vi "Begin.vi"(8 "error in":errorcluster) -> (0 "error out":errorcluster)   [LabVIEW 2016]
doc: "Called before other user functions, this VI is expected to open initial I/O refnums, load in file data, and do all program initialization. Notice that the <B>error out</B> terminal is simply used for data flow. Wiring it to other structures or subVIs ensures that this VI runs first."
uses:
  <vilib>/Rock Robotics/WPI/DriverStation/WPI_DriverStationRobotMode2.ctl
  <vilib>/Rock Robotics/WPI/Joystick/WPI_JoystickDeviceEnum.ctl
  <vilib>/Rock Robotics/WPI/ThirdParty/CanMotor/TalonSRX/WPI_CANTalonSRX_APIControlMode.ctl
  <vilib>/Rock Robotics/SystemInterfaces/DIO/FPGA_DIOPWMChannel.ctl
  <vilib>/Rock Robotics/WPI/Solenoid/WPI_SolenoidChannel.ctl
  <vilib>/Rock Robotics/WPI/ThirdParty/CanMotor/TalonSRX/WPI_CANTalonSRX_APIFeedbackSelect.ctl
  <vilib>/Rock Robotics/WPI/SafetyOutput/WPI_SafetyOutputConfigMenu.ctl
  <vilib>/Rock Robotics/SystemInterfaces/DIO/FPGA_DIOChannel.ctl
  <vilib>/Rock Robotics/SystemInterfaces/spilib/spi_bus.ctl
  Robot Global Data.vi
  <vilib>/Rock Robotics/Network Tables/NT Write String Array.vi
  <vilib>/Rock Robotics/WPI/MotorControl/WPI_MotorControlOpen VictorSP.vi
  <vilib>/Rock Robotics/WPI/Solenoid/WPI_SolenoidOpenDouble.vi
  <vilib>/Rock Robotics/WPI/Switch/WPI_SwitchOpenLimit.vi
  <vilib>/Rock Robotics/Network Tables/NT Write Boolean.vi
  <vilib>/Rock Robotics/WPI/Gyro/WPI_GyroXRS450_SPI_Open.vi
  <vilib>/Rock Robotics/WPI/Counter/WPI_CounterDigitalInputToDigitalSource.vi
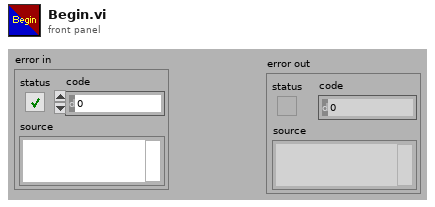
[diagram p1: front panel]
types:
  T1 = typedef "FPGA_DIOChannel.ctl" = enum8{"DIO 0", "DIO 1", "DIO 2", "DIO 3", "DIO 4", "DIO 5", "DIO 6", "DIO 7", "DIO 8", "DIO 9", "DIO MXP 0", "DIO MXP 1", "DIO MXP 2", "DIO MXP 3", "DIO MXP 4", "DIO MXP 5", "DIO MXP 6", "DIO MXP 7", "DIO MXP 8", "DIO MXP 9", "DIO MXP 10", "DIO MXP 11", "DIO MXP 12", "DIO MXP 13", "DIO MXP 14", "DIO MXP 15", "SPI Port CS1", "SPI Port CS2", "SPI Port CS3", "SPI Port MISO", "SPI Port MOSI", "Invalid"}
  T2 = typedef "spi_bus.ctl" = enum16{"SPI On-Board, CS0", "SPI On-Board, CS1", "SPI On-Board, CS2", "SPI On-Board, CS3", "SPI MXP", "Invalid"}
  T3 = typedef "WPI_CANTalonSRX_APIControlMode.ctl" = enum8{"Percent VBus", "Speed", "Position", "Slave", "Unchanged / Invalid", "Voltage Compensation", "Current", "Motion Profile", "Motion Magic"}
  T4 = typedef "WPI_JoystickDeviceEnum.ctl" = enum16{"USB 0", "USB 1", "USB 2", "USB 3", "USB 4", "USB 5"}
  T5 = typedef "WPI_SafetyOutputConfigMenu.ctl" = enum16{"Enable", "Disable"}
  T6 = typedef "WPI_SolenoidChannel.ctl" = enum8{"Solenoid 0", "Solenoid 1", "Solenoid 2", "Solenoid 3", "Solenoid 4", "Solenoid 5", "Solenoid 6", "Solenoid 7", "Invalid"}
  T7 = typedef "WPI_CANTalonSRX_APIFeedbackSelect.ctl" = enum16{"Digital Quadrature Encoder", "Analog Potentiometer", "Analog Encoder", "Count on Quad-A (Rising-Edge)", "Count on Quad-A (Falling-Edge)", "CTR Magnetic Enc (Absolute)", "CTR Magnetic Enc (Relative)", "Pulse Width"}
  T8 = typedef "FPGA_DIOPWMChannel.ctl" = enum8{"PWM 0", "PWM 1", "PWM 2", "PWM 3", "PWM 4", "PWM 5", "PWM 6", "PWM 7", "PWM 8", "PWM 9", "PWM MXP 0", "PWM MXP 1", "PWM MXP 2", "PWM MXP 3", "PWM MXP 4", "PWM MXP 5", "PWM MXP 6", "PWM MXP 7", "PWM MXP 8", "PWM MXP 9", "Invalid"}
  T9 = typedef "WPI_DriverStationRobotMode2.ctl" = enum16{"Autonomous Disabled", "Autonomous Enabled", "Teleop Disabled", "Teleop Enabled", "Disconnected", "Finish", "Test Disabled", "Test Enabled", "Emergency Stopped"}
  T10 = typedef "WPI_JoystickDevRef.ctl" = cluster{"Device":T4}
  T11 = typedef "WPI_DigitalInputDevRef.ctl" = cluster{"DevStatus":errorcluster, "DIO Channel":T1}
  T12 = typedef "FPGA_CounterEncoderSourceConvertionLVSourceType.ctl" = cluster{"DevStatus":errorcluster, "AnalogTriggerMode?":bool, "DigitalMode":cluster{"DIO Channel":T13}, "AnalogTriggerMode":cluster{"AnalogTriggerIndex":T14, "OutputType":T15}}
  T13 = typedef "FPGA_DIODigitalSourceChannel.ctl" = enum8{"DIO 0", "DIO 1", "DIO 2", "DIO 3", "DIO 4", "DIO 5", "DIO 6", "DIO 7", "DIO 8", "DIO 9", "DIO MXP 0", "DIO MXP 1", "DIO MXP 2", "DIO MXP 3", "DIO MXP 4", "DIO MXP 5", "DIO MXP 6", "DIO MXP 7", "DIO MXP 8", "DIO MXP 9", "DIO MXP 10", "DIO MXP 11", "DIO MXP 12", "DIO MXP 13", "DIO MXP 14", "DIO MXP 15", "Disabled"}
  T14 = typedef "FPGA_AnalogTriggerIndex.ctl" = enum8{"Trig 0", "Trig 1", "Trig 2", "Trig 3", "Trig 4", "Trig 5", "Trig 6", "Trig 7", "Invalid"}
  T15 = typedef "FPGA_AnalogTriggerOutType.ctl" = enum16{"InWindow", "TriggerState", "Rising", "Falling"}
  T16 = typedef "WPI_EncoderDevRef.ctl" = cluster{"DevStatus":errorcluster, "EncoderIndex":T17, "CounterIndex":T18, "DistancePerCount":dbl, "Decoding Type":T19}
  T17 = typedef "FPGA_EncoderIdx.ctl" = enum8{"Enc 0", "Enc 1", "Enc 2", "Enc 3", "Enc 4", "Enc 5", "Enc 6", "Enc 7", "Invalid"}
  T18 = typedef "FPGA_CounterCtrSystemIndex.ctl" = enum8{"Ctr 0", "Ctr 1", "Ctr 2", "Ctr 3", "Ctr 4", "Ctr 5", "Ctr 6", "Ctr 7", "Invalid"}
  T19 = typedef "WPI_EncoderType.ctl" = enum16{"1x", "2x", "4x"}
  T20 = typedef "WPI_SolenoidDevRef.ctl" = cluster{"DevStatus":errorcluster, "Pneumatics Control Module":u8, "Forward Solenoid Channel":T6, "Reverse Solenoid Channel":T6}
  T21 = typedef "WPI_MotorControlDeviceRef.ctl" = cluster{"DeviceStatus":errorcluster, "Type":T22, "PWM":cluster{"PWM Channel":T8, "DeadBand":T23}, "CAN":cluster{"Device Number":u8, "SetOutput VI Ref":variant, "GetOutput VI Ref":variant, "Enable VI Ref":variant, "Disable VI Ref":variant, "Data":variant}, "Invert":bool}
  T22 = typedef "WPI_MotorControlType.ctl" = enum16{"PWM", "CAN"}
  T23 = typedef "WPI_PWMDeadband.ctl" = cluster{"Name":string, "maxPositivePwm":i32, "minPositivePwm":i32, "centerPwm":i32, "maxNegativePwm":i32, "minNegativePwm":i32, "angularRange":u16}
  T24 = typedef "WPI_SwitchDevRef.ctl" = cluster{"DevStatus":errorcluster, "DIO Channel":T1, "CntIndex":T18, "Normally Closed":bool}
  T25 = typedef "WPI_GyroDevRef.ctl" = cluster{"DevStatus":errorcluster, "Analog Channel":T26, "Offset":dbl, "Gain (VoltsPerDegree/Second)":dbl, "Gyro Type":enum16{"Analog", "XRS450"}, "Handle":i32, "SPI Bus":T2, "Device Found":bool, "Sample Rate":dbl, "Calibrate On Open":bool}
  T26 = typedef "FPGA_AIChannel.ctl" = enum8{"AI 0", "AI 1", "AI 2", "AI 3", "AI MXP 0", "AI MXP 1", "AI MXP 2", "AI MXP 3", "Invalid"}
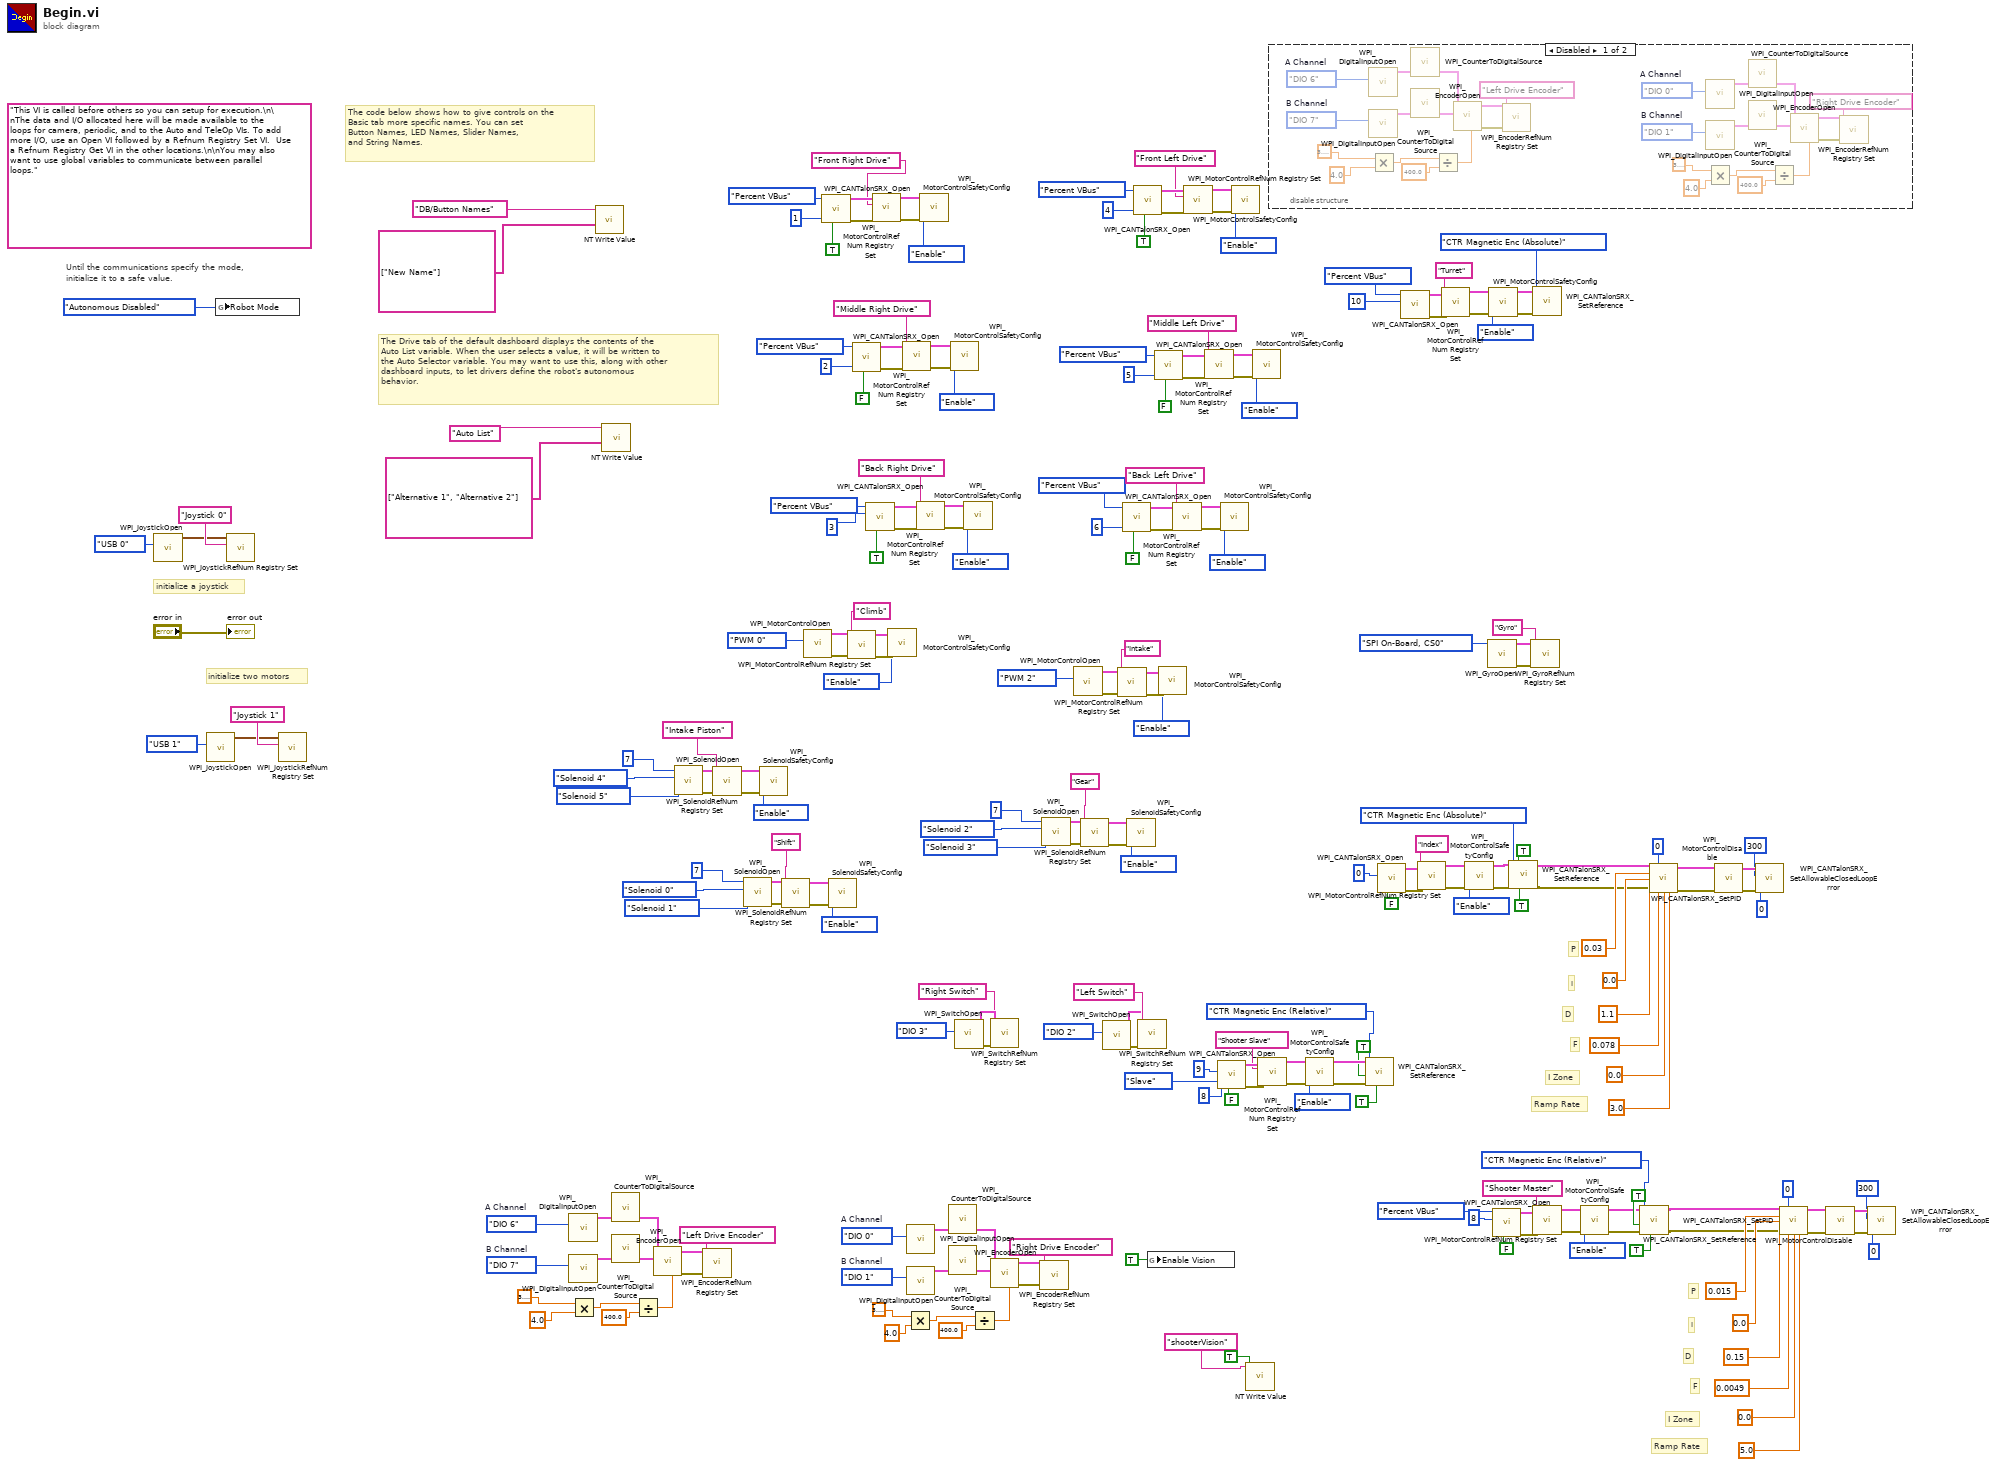
[diagram p0: block diagram]
diagram:
  w19 = FPGA_DIOChannel."DIO 1"  # B Channel
  w18 = FPGA_DIOChannel."DIO 0"  # A Channel
  w28 = FPGA_DIOChannel."DIO 7"  # B Channel
  w27 = FPGA_DIOChannel."DIO 6"  # A Channel
  (unwired) "This VI is called before others so you can setup for execution.\n\nThe data and I/O allocated here will be made available to the loops for camera, periodic, and to the Auto and TeleOp VIs. To add more I/O, use an Open VI followed by a Refnum Registry Set VI.  Use a Refnum Registry Get VI in the other locations.\n\nYou may also want to use global variables to communicate between parallel loops."
  # "Ramp Rate"
  # "I Zone"
  # "F"
  # "D"
  # "I"
  # "P"
  # "Ramp Rate"
  # "I Zone"
  # "F"
  # "D"
  # "I"
  # "P"
  # "initialize two motors"
  # "The Drive tab of the default dashboard displays the contents of the\nAuto List variable. When the user selects a value, it will be written to\nthe Auto Selector variable. You may want to use this, along with other\ndashboard inputs, to let drivers define the robot's autonomous\nbehavior."
  # "The code below shows how to give controls on the\nBasic tab more specific names. You can set\nButton Names, LED Names, Slider Names,\nand String Names."
  # "initialize a joystick"
  # "Until the communications specify the mode,\ninitialize it to a safe value."
  n1 = call <vilib>:"WPI_JoystickOpen.vi"("JoystickDevice"=WPI_JoystickDeviceEnum."USB 0") -> ("JoystickDevRef"=w231:T10)  [unwired: 10 in]
  n2 = call <vilib>:"WPI_JoystickOpen.vi"("JoystickDevice"=WPI_JoystickDeviceEnum."USB 1") -> ("JoystickDevRef"=w78:T10)  [unwired: 10 in]
  n3 = global write "Robot Global Data.vi" "Robot Mode"(WPI_DriverStationRobotMode2."Autonomous Disabled" ("Robot Mode")) -> ()
  n4 = call <vilib>:"WPI_JoystickRefNum Registry Set.vi"("refnum name"="Joystick 0", "JoystickDevRef"=w231) -> ()  [unwired: 8 in, 2 out]
  n5 = call <vilib>:"WPI_JoystickRefNum Registry Set.vi"("refnum name"="Joystick 1", "JoystickDevRef"=w78) -> ()  [unwired: 8 in, 2 out]
  n6 = call <vilib>:"WPI_DigitalInputOpen.vi"("DIO Channel"=w27) -> ("DigitalInputDevRef"=w24:T11)  [unwired: 1 in, 9 out]
  n7 = call <vilib>:"WPI_DigitalInputOpen.vi"("DIO Channel"=w28) -> ("DigitalInputDevRef"=w25:T11)  [unwired: 1 in, 9 out]
  n8 = Multiply(x=3.141592653589793, y=4.0) -> (x*y=w3:dbl)
  n9 = call-poly <vilib>:"NT Write Value.vi"("String Array"=string[] ["New Name"], "Name"="DB/Button Names") -> ()  [unwired: 9 in, 1 out]
  n10 = call-poly <vilib>:"NT Write Value.vi"("String Array"=string[] ["Alternative 1", "Alternative 2"], "Name"="Auto List") -> ()  [unwired: 9 in, 1 out]
  n11 = call-poly <vilib>:"WPI_CounterToDigitalSource.vi"("DigitalInputDevRef"=w24) -> ("Digital Source"=w23:T12)  [unwired: 6 out]
  n12 = call-poly <vilib>:"WPI_CounterToDigitalSource.vi"("DigitalInputDevRef"=w25) -> ("Digital Source"=w26:T12)  [unwired: 6 out]
  n13 = Divide(x=w3, y=400.0) -> (x/y=w1:dbl)
  n14 = call <vilib>:"WPI_EncoderOpen.vi"("DistancePerCount"=w1, "BSource"=w26, "ASource"=w23) -> ("error out"=w22:errorcluster, "EncoderDevRef"=w21:T16)  [unwired: 5 in, 2 out]
  n15 = call-poly <vilib>:"WPI_SolenoidOpen.vi"("Reverse Solenoid Channel"=WPI_SolenoidChannel."Solenoid 5", "Forward Solenoid Channel"=WPI_SolenoidChannel."Solenoid 4", "Pneumatics Control Module (0)"=u8 7) -> ("error out"=w155:errorcluster, "SolenoidDevRef"=w154:T20)  [unwired: 7 in]
  n16 = call <vilib>:"WPI_EncoderRefNum Registry Set.vi"("error in (no error)"=w22, "refnum name"="Left Drive Encoder", "EncoderDevRef"=w21) -> ()  [unwired: 7 in, 2 out]
  n17 = call <vilib>:"WPI_SolenoidRefNum Registry Set.vi"("error in (no error)"=w155, "refnum name"="Intake Piston", "SolenoidDevRef"=w154) -> ("error out"=w152:errorcluster, "SolenoidDevRef"=w151:T20)  [unwired: 7 in]
  n18 = call-poly <vilib>:"WPI_SolenoidOpen.vi"("Reverse Solenoid Channel"=WPI_SolenoidChannel."Solenoid 1", "Forward Solenoid Channel"=WPI_SolenoidChannel."Solenoid 0", "Pneumatics Control Module (0)"=u8 7) -> ("error out"=w85:errorcluster, "SolenoidDevRef"=w84:T20)  [unwired: 7 in]
  n19 = call <vilib>:"WPI_SolenoidSafetyConfig.vi"("error in (no error)"=w152, "mode"=WPI_SafetyOutputConfigMenu."Enable", "SolenoidDevRef"=w151) -> ()  [unwired: 7 in, 2 out]
  n20 = call <vilib>:"WPI_SolenoidRefNum Registry Set.vi"("error in (no error)"=w85, "refnum name"="Shift", "SolenoidDevRef"=w84) -> ("error out"=w82:errorcluster, "SolenoidDevRef"=w81:T20)  [unwired: 7 in]
  n21 = call-poly <vilib>:"WPI_MotorControlOpen.vi"("PWM Channel"=FPGA_DIOPWMChannel."PWM 0") -> ("error out"=w170:errorcluster, "MotorControlDeviceRef"=w169:T21)  [unwired: 9 in]
  n22 = call <vilib>:"WPI_CANTalonSRX_Open.vi"("Invert"=TRUE, "Device Number"=u8 1, "Control Mode"=WPI_CANTalonSRX_APIControlMode."Percent VBus") -> ("error out"=w186:errorcluster, "CAN Talon SRX Ref"=w185:T21)  [unwired: 7 in]
  n23 = call <vilib>:"WPI_SolenoidSafetyConfig.vi"("error in (no error)"=w82, "mode"=WPI_SafetyOutputConfigMenu."Enable", "SolenoidDevRef"=w81) -> ()  [unwired: 7 in, 2 out]
  n24 = call <vilib>:"WPI_MotorControlRefNum Registry Set.vi"("error in (no error)"=w170, "refnum name"="Climb", "MotorControlDevRef"=w169) -> ("error out"=w166:errorcluster, "MotorControlDevRef"=w165:T21)  [unwired: 7 in]
  n25 = call <vilib>:"WPI_CANTalonSRX_Open.vi"("Invert"=FALSE, "Device Number"=u8 2, "Control Mode"=WPI_CANTalonSRX_APIControlMode."Percent VBus") -> ("error out"=w221:errorcluster, "CAN Talon SRX Ref"=w220:T21)  [unwired: 7 in]
  n26 = call <vilib>:"WPI_CANTalonSRX_Open.vi"("Invert"=TRUE, "Device Number"=u8 3, "Control Mode"=WPI_CANTalonSRX_APIControlMode."Percent VBus") -> ("error out"=w204:errorcluster, "CAN Talon SRX Ref"=w203:T21)  [unwired: 7 in]
  n27 = call <vilib>:"WPI_MotorControlRefNum Registry Set.vi"("error in (no error)"=w186, "refnum name"="Front Right Drive", "MotorControlDevRef"=w185) -> ("error out"=w184:errorcluster, "MotorControlDevRef"=w183:T21)  [unwired: 7 in]
  n28 = call <vilib>:"WPI_MotorControlSafetyConfig.vi"("error in (no error)"=w166, "mode"=WPI_SafetyOutputConfigMenu."Enable", "MotorControlDevRef"=w165) -> ()  [unwired: 7 in, 2 out]
  n29 = call <vilib>:"WPI_MotorControlRefNum Registry Set.vi"("error in (no error)"=w221, "refnum name"="Middle Right Drive", "MotorControlDevRef"=w220) -> ("error out"=w219:errorcluster, "MotorControlDevRef"=w218:T21)  [unwired: 7 in]
  n30 = call <vilib>:"WPI_DigitalInputOpen.vi"("DIO Channel"=w18) -> ("DigitalInputDevRef"=w15:T11)  [unwired: 1 in, 9 out]
  n31 = call <vilib>:"WPI_DigitalInputOpen.vi"("DIO Channel"=w19) -> ("DigitalInputDevRef"=w16:T11)  [unwired: 1 in, 9 out]
  n32 = Multiply(x=3.141592653589793, y=4.0) -> (x*y=w8:dbl)
  n33 = call <vilib>:"WPI_MotorControlRefNum Registry Set.vi"("error in (no error)"=w204, "refnum name"="Back Right Drive", "MotorControlDevRef"=w203) -> ("error out"=w202:errorcluster, "MotorControlDevRef"=w201:T21)  [unwired: 7 in]
  n34 = call <vilib>:"WPI_MotorControlSafetyConfig.vi"("error in (no error)"=w184, "mode"=WPI_SafetyOutputConfigMenu."Enable", "MotorControlDevRef"=w183) -> ()  [unwired: 7 in, 2 out]
  n35 = call-poly <vilib>:"WPI_CounterToDigitalSource.vi"("DigitalInputDevRef"=w15) -> ("Digital Source"=w14:T12)  [unwired: 6 out]
  n36 = call-poly <vilib>:"WPI_CounterToDigitalSource.vi"("DigitalInputDevRef"=w16) -> ("Digital Source"=w17:T12)  [unwired: 6 out]
  n37 = call <vilib>:"WPI_MotorControlSafetyConfig.vi"("error in (no error)"=w219, "mode"=WPI_SafetyOutputConfigMenu."Enable", "MotorControlDevRef"=w218) -> ()  [unwired: 7 in, 2 out]
  n38 = call-poly <vilib>:"WPI_SwitchOpen.vi"("DIO Channel"=FPGA_DIOChannel."DIO 3") -> ("error out"=w76:errorcluster, "SwitchDevRef"=w75:T24)  [unwired: 9 in]
  n39 = call <vilib>:"WPI_MotorControlSafetyConfig.vi"("error in (no error)"=w202, "mode"=WPI_SafetyOutputConfigMenu."Enable", "MotorControlDevRef"=w201) -> ()  [unwired: 7 in, 2 out]
  n40 = Divide(x=w8, y=400.0) -> (x/y=w6:dbl)
  n41 = call <vilib>:"WPI_SwitchRefNum Registry Set.vi"("error in (no error)"=w76, "refnum name"="Right Switch", "SwitchDevRef"=w75) -> ()  [unwired: 7 in, 2 out]
  n42 = call <vilib>:"WPI_EncoderOpen.vi"("DistancePerCount"=w6, "BSource"=w17, "ASource"=w14) -> ("error out"=w13:errorcluster, "EncoderDevRef"=w12:T16)  [unwired: 5 in, 2 out]
  n43 = call <vilib>:"WPI_EncoderRefNum Registry Set.vi"("error in (no error)"=w13, "refnum name"="Right Drive Encoder", "EncoderDevRef"=w12) -> ()  [unwired: 7 in, 2 out]
  n44 = call-poly <vilib>:"WPI_SolenoidOpen.vi"("Reverse Solenoid Channel"=WPI_SolenoidChannel."Solenoid 3", "Forward Solenoid Channel"=WPI_SolenoidChannel."Solenoid 2", "Pneumatics Control Module (0)"=u8 7) -> ("error out"=w142:errorcluster, "SolenoidDevRef"=w143:T20)  [unwired: 7 in]
  n45 = call-poly <vilib>:"WPI_MotorControlOpen.vi"("PWM Channel"=FPGA_DIOPWMChannel."PWM 2") -> ("error out"=w164:errorcluster, "MotorControlDeviceRef"=w163:T21)  [unwired: 9 in]
  n46 = call <vilib>:"WPI_SolenoidRefNum Registry Set.vi"("error in (no error)"=w142, "refnum name"="Gear", "SolenoidDevRef"=w143) -> ("error out"=w145:errorcluster, "SolenoidDevRef"=w146:T20)  [unwired: 7 in]
  n47 = call-poly <vilib>:"WPI_SwitchOpen.vi"("DIO Channel"=FPGA_DIOChannel."DIO 2") -> ("error out"=w69:errorcluster, "SwitchDevRef"=w70:T24)  [unwired: 9 in]
  n48 = call <vilib>:"WPI_MotorControlRefNum Registry Set.vi"("error in (no error)"=w164, "refnum name"="Intake", "MotorControlDevRef"=w163) -> ("error out"=w160:errorcluster, "MotorControlDevRef"=w159:T21)  [unwired: 7 in]
  n49 = call <vilib>:"WPI_CANTalonSRX_Open.vi"("Invert"=FALSE, "Device Number"=u8 6, "Control Mode"=WPI_CANTalonSRX_APIControlMode."Percent VBus") -> ("error out"=w196:errorcluster, "CAN Talon SRX Ref"=w195:T21)  [unwired: 7 in]
  n50 = call <vilib>:"WPI_SolenoidSafetyConfig.vi"("error in (no error)"=w145, "mode"=WPI_SafetyOutputConfigMenu."Enable", "SolenoidDevRef"=w146) -> ()  [unwired: 7 in, 2 out]
  n51 = call <vilib>:"WPI_CANTalonSRX_Open.vi"("Invert"=TRUE, "Device Number"=u8 4, "Control Mode"=WPI_CANTalonSRX_APIControlMode."Percent VBus") -> ("error out"=w212:errorcluster, "CAN Talon SRX Ref"=w211:T21)  [unwired: 7 in]
  n52 = call <vilib>:"WPI_SwitchRefNum Registry Set.vi"("error in (no error)"=w69, "refnum name"="Left Switch", "SwitchDevRef"=w70) -> ()  [unwired: 7 in, 2 out]
  n53 = global write "Robot Global Data.vi" "Enable Vision"(TRUE ("Enable Vision")) -> ()
  n54 = call <vilib>:"WPI_CANTalonSRX_Open.vi"("Invert"=FALSE, "Device Number"=u8 5, "Control Mode"=WPI_CANTalonSRX_APIControlMode."Percent VBus") -> ("error out"=w178:errorcluster, "CAN Talon SRX Ref"=w173:T21)  [unwired: 7 in]
  n55 = call <vilib>:"WPI_MotorControlSafetyConfig.vi"("error in (no error)"=w160, "mode"=WPI_SafetyOutputConfigMenu."Enable", "MotorControlDevRef"=w159) -> ()  [unwired: 7 in, 2 out]
  n56 = call <vilib>:"WPI_MotorControlRefNum Registry Set.vi"("error in (no error)"=w196, "refnum name"="Back Left Drive", "MotorControlDevRef"=w195) -> ("error out"=w194:errorcluster, "MotorControlDevRef"=w193:T21)  [unwired: 7 in]
  n57 = call <vilib>:"WPI_MotorControlRefNum Registry Set.vi"("error in (no error)"=w212, "refnum name"="Front Left Drive", "MotorControlDevRef"=w211) -> ("error out"=w210:errorcluster, "MotorControlDevRef"=w209:T21)  [unwired: 7 in]
  n58 = call <vilib>:"WPI_MotorControlRefNum Registry Set.vi"("error in (no error)"=w178, "refnum name"="Middle Left Drive", "MotorControlDevRef"=w173) -> ("error out"=w177:errorcluster, "MotorControlDevRef"=w176:T21)  [unwired: 7 in]
  n59 = call <vilib>:"WPI_CANTalonSRX_Open.vi"("Invert"=FALSE, "Master Device Number"=u8 8, "Device Number"=u8 9, "Control Mode"=WPI_CANTalonSRX_APIControlMode."Slave") -> ("error out"=w117:errorcluster, "CAN Talon SRX Ref"=w118:T21)  [unwired: 6 in]
  n60 = call <vilib>:"WPI_MotorControlSafetyConfig.vi"("error in (no error)"=w194, "mode"=WPI_SafetyOutputConfigMenu."Enable", "MotorControlDevRef"=w193) -> ()  [unwired: 7 in, 2 out]
  n61 = call <vilib>:"WPI_MotorControlSafetyConfig.vi"("error in (no error)"=w210, "mode"=WPI_SafetyOutputConfigMenu."Enable", "MotorControlDevRef"=w209) -> ()  [unwired: 7 in, 2 out]
  n62 = call-poly <vilib>:"NT Write Value.vi"("Boolean"=TRUE, "Name"="shooterVision") -> ()  [unwired: 9 in, 1 out]
  n63 = call <vilib>:"WPI_MotorControlSafetyConfig.vi"("error in (no error)"=w177, "mode"=WPI_SafetyOutputConfigMenu."Enable", "MotorControlDevRef"=w176) -> ()  [unwired: 7 in, 2 out]
  n64 = call <vilib>:"WPI_MotorControlRefNum Registry Set.vi"("error in (no error)"=w117, "refnum name"="Shooter Slave", "MotorControlDevRef"=w118) -> ("error out"=w113:errorcluster, "MotorControlDevRef"=w116:T21)  [unwired: 7 in]
  n65 = disable-structure shown="Disabled" {
    frame Disabled {
      w252 = FPGA_DIOChannel."DIO 1"  # B Channel
      w251 = FPGA_DIOChannel."DIO 0"  # A Channel
      w261 = FPGA_DIOChannel."DIO 7"  # B Channel
      w260 = FPGA_DIOChannel."DIO 6"  # A Channel
      n66 = call <vilib>:"WPI_DigitalInputOpen.vi"("DIO Channel"=w260) -> ("DigitalInputDevRef"=w257:T11)  [unwired: 1 in, 9 out]
      n67 = call <vilib>:"WPI_DigitalInputOpen.vi"("DIO Channel"=w261) -> ("DigitalInputDevRef"=w258:T11)  [unwired: 1 in, 9 out]
      n68 = Multiply(x=3.141592653589793, y=4.0) -> (x*y=w236:dbl)
      n69 = call-poly <vilib>:"WPI_CounterToDigitalSource.vi"("DigitalInputDevRef"=w257) -> ("Digital Source"=w256:T12)  [unwired: 6 out]
      n70 = call-poly <vilib>:"WPI_CounterToDigitalSource.vi"("DigitalInputDevRef"=w258) -> ("Digital Source"=w259:T12)  [unwired: 6 out]
      n71 = Divide(x=w236, y=400.0) -> (x/y=w234:dbl)
      n72 = call <vilib>:"WPI_EncoderOpen.vi"("DistancePerCount"=w234, "BSource"=w259, "ASource"=w256) -> ("error out"=w255:errorcluster, "EncoderDevRef"=w254:T16)  [unwired: 5 in, 2 out]
      n73 = call <vilib>:"WPI_EncoderRefNum Registry Set.vi"("error in (no error)"=w255, "refnum name"="Left Drive Encoder", "EncoderDevRef"=w254) -> ()  [unwired: 7 in, 2 out]
      n74 = call <vilib>:"WPI_DigitalInputOpen.vi"("DIO Channel"=w251) -> ("DigitalInputDevRef"=w248:T11)  [unwired: 1 in, 9 out]
      n75 = call <vilib>:"WPI_DigitalInputOpen.vi"("DIO Channel"=w252) -> ("DigitalInputDevRef"=w249:T11)  [unwired: 1 in, 9 out]
      n76 = Multiply(x=3.141592653589793, y=4.0) -> (x*y=w241:dbl)
      n77 = call-poly <vilib>:"WPI_CounterToDigitalSource.vi"("DigitalInputDevRef"=w248) -> ("Digital Source"=w247:T12)  [unwired: 6 out]
      n78 = call-poly <vilib>:"WPI_CounterToDigitalSource.vi"("DigitalInputDevRef"=w249) -> ("Digital Source"=w250:T12)  [unwired: 6 out]
      n79 = Divide(x=w241, y=400.0) -> (x/y=w239:dbl)
      n80 = call <vilib>:"WPI_EncoderOpen.vi"("DistancePerCount"=w239, "BSource"=w250, "ASource"=w247) -> ("error out"=w246:errorcluster, "EncoderDevRef"=w245:T16)  [unwired: 5 in, 2 out]
      n81 = call <vilib>:"WPI_EncoderRefNum Registry Set.vi"("error in (no error)"=w246, "refnum name"="Right Drive Encoder", "EncoderDevRef"=w245) -> ()  [unwired: 7 in, 2 out]
    }
    frame Enabled {
    }
  }
  n82 = call <vilib>:"WPI_MotorControlSafetyConfig.vi"("error in (no error)"=w113, "mode"=WPI_SafetyOutputConfigMenu."Enable", "MotorControlDevRef"=w116) -> ("error out"=w120:errorcluster, "MotorControlDevRef"=w124:T21)  [unwired: 7 in]
  n83 = call <vilib>:"WPI_CANTalonSRX_SetReference.vi"("Reverse Closed-Loop Output"=TRUE, "error in (no error)"=w120, "Reverse Feedback Sensor"=TRUE, "Feedback Reference"=WPI_CANTalonSRX_APIFeedbackSelect."CTR Magnetic Enc (Relative)", "CAN Talon SRX Ref"=w124) -> ()  [unwired: 5 in, 2 out]
  n84 = call <vilib>:"WPI_CANTalonSRX_Open.vi"("Invert"=FALSE, "Device Number"=u8 0) -> ("error out"=w107:errorcluster, "CAN Talon SRX Ref"=w106:T21)  [unwired: 8 in]
  n85 = call <vilib>:"WPI_CANTalonSRX_Open.vi"("Device Number"=u8 10, "Control Mode"=WPI_CANTalonSRX_APIControlMode."Percent VBus") -> ("error out"=w94:errorcluster, "CAN Talon SRX Ref"=w93:T21)  [unwired: 8 in]
  n86 = call <vilib>:"WPI_MotorControlRefNum Registry Set.vi"("error in (no error)"=w107, "refnum name"="Index", "MotorControlDevRef"=w106) -> ("error out"=w112:errorcluster, "MotorControlDevRef"=w108:T21)  [unwired: 7 in]
  n87 = call <vilib>:"WPI_MotorControlRefNum Registry Set.vi"("error in (no error)"=w94, "refnum name"="Turret", "MotorControlDevRef"=w93) -> ("error out"=w99:errorcluster, "MotorControlDevRef"=w95:T21)  [unwired: 7 in]
  n88 = call <vilib>:"WPI_MotorControlSafetyConfig.vi"("error in (no error)"=w112, "mode"=WPI_SafetyOutputConfigMenu."Enable", "MotorControlDevRef"=w108) -> ("error out"=w104:errorcluster, "MotorControlDevRef"=w100:T21)  [unwired: 7 in]
  n89 = call-poly <vilib>:"WPI_GyroOpen.vi"("SPI Bus"=spi_bus."SPI On-Board, CS0") -> ("error out"=w32:errorcluster, "GyroDevRef"=w31:T25)  [unwired: 9 in]
  n90 = call <vilib>:"WPI_MotorControlSafetyConfig.vi"("error in (no error)"=w99, "mode"=WPI_SafetyOutputConfigMenu."Enable", "MotorControlDevRef"=w95) -> ("error out"=w90:errorcluster, "MotorControlDevRef"=w91:T21)  [unwired: 7 in]
  n91 = call <vilib>:"WPI_CANTalonSRX_Open.vi"("Invert"=FALSE, "Device Number"=u8 8, "Control Mode"=WPI_CANTalonSRX_APIControlMode."Percent VBus") -> ("error out"=w134:errorcluster, "CAN Talon SRX Ref"=w133:T21)  [unwired: 7 in]
  n92 = call <vilib>:"WPI_CANTalonSRX_SetReference.vi"("Reverse Closed-Loop Output"=TRUE, "error in (no error)"=w104, "Reverse Feedback Sensor"=TRUE, "Feedback Reference"=WPI_CANTalonSRX_APIFeedbackSelect."CTR Magnetic Enc (Absolute)", "CAN Talon SRX Ref"=w100) -> ("error out"=w39:errorcluster, "CAN Talon SRX Ref"=w40:T21)  [unwired: 5 in]
  n93 = call <vilib>:"WPI_GyroRefNum Registry Set.vi"("error in (no error)"=w32, "refnum name"="Gyro", "GyroDevRef"=w31) -> ()  [unwired: 7 in, 2 out]
  n94 = call <vilib>:"WPI_CANTalonSRX_SetReference.vi"("error in (no error)"=w90, "Feedback Reference"=WPI_CANTalonSRX_APIFeedbackSelect."CTR Magnetic Enc (Absolute)", "CAN Talon SRX Ref"=w91) -> ()  [unwired: 7 in, 2 out]
  n95 = call <vilib>:"WPI_MotorControlRefNum Registry Set.vi"("error in (no error)"=w134, "refnum name"="Shooter Master", "MotorControlDevRef"=w133) -> ("error out"=w138:errorcluster, "MotorControlDevRef"=w135:T21)  [unwired: 7 in]
  n96 = call <vilib>:"WPI_MotorControlSafetyConfig.vi"("error in (no error)"=w138, "mode"=WPI_SafetyOutputConfigMenu."Enable", "MotorControlDevRef"=w135) -> ("error out"=w131:errorcluster, "MotorControlDevRef"=w127:T21)  [unwired: 7 in]
  n97 = call <vilib>:"WPI_CANTalonSRX_SetReference.vi"("Reverse Closed-Loop Output"=TRUE, "error in (no error)"=w131, "Reverse Feedback Sensor"=TRUE, "Feedback Reference"=WPI_CANTalonSRX_APIFeedbackSelect."CTR Magnetic Enc (Relative)", "CAN Talon SRX Ref"=w127) -> ("error out"=w54:errorcluster, "CAN Talon SRX Ref"=w55:T21)  [unwired: 5 in]
  n98 = call <vilib>:"WPI_CANTalonSRX_SetPID.vi"("CAN Talon SRX Ref"=w40, "Parameter Slot"=u8 0, "P"=0.03, "I"=0.0, "D"=1.1 ("P"), "error in (no error)"=w39, "F"=0.078 ("I"), "I Zone"=0.0 ("P"), "Ramp Rate"=3.0 ("I")) -> ("CAN Talon SRX Ref"=w52:T21, "error out"=w51:errorcluster)  [unwired: 5 in]
  n99 = call <vilib>:"WPI_MotorControlDisable.vi"("error in (no error)"=w51, "MotorControlDevRef"=w52) -> ("error out"=w50:errorcluster, "MotorControlDevRef"=w49:T21)  [unwired: 8 in]
  n100 = call <vilib>:"WPI_CANTalonSRX_SetAllowableClosedLoopError.vi"("error in (no error)"=w50, "Parameter Slot"=u8 0, "Allowable Closed-Loop Error"=u16 300, "CAN Talon SRX Ref"=w49) -> ()  [unwired: 6 in, 2 out]
  n101 = call <vilib>:"WPI_CANTalonSRX_SetPID.vi"("CAN Talon SRX Ref"=w55, "Parameter Slot"=u8 0, "P"=0.015, "I"=0.0, "D"=0.15 ("P"), "error in (no error)"=w54, "F"=0.0049 ("I"), "I Zone"=0.0 ("P"), "Ramp Rate"=5.0 ("I")) -> ("CAN Talon SRX Ref"=w67:T21, "error out"=w66:errorcluster)  [unwired: 5 in]
  n102 = call <vilib>:"WPI_MotorControlDisable.vi"("error in (no error)"=w66, "MotorControlDevRef"=w67) -> ("error out"=w65:errorcluster, "MotorControlDevRef"=w64:T21)  [unwired: 8 in]
  n103 = call <vilib>:"WPI_CANTalonSRX_SetAllowableClosedLoopError.vi"("error in (no error)"=w65, "Parameter Slot"=u8 0, "Allowable Closed-Loop Error"=u16 300, "CAN Talon SRX Ref"=w64) -> ()  [unwired: 6 in, 2 out]
  "error out" <- "error in"
